vi "FillClassFamTree.vi"(7 "référence":refnum<vi>, 8 "ErrorIn(No Error)":errorcluster caption="entrée d'erreur (pas d'erreur)", 9 "LdClassArr":string[](array[string]), 10 "LdNameArr":string[](array[string]), 11 "SelectedClass":string) -> (0 "sortie d'erreur":errorcluster, 1 "Text":string[][](array[string]), 2 "Functions":string[][](array[string]), 3 "Classes":string[][](array[string]))   [LabVIEW 2019]
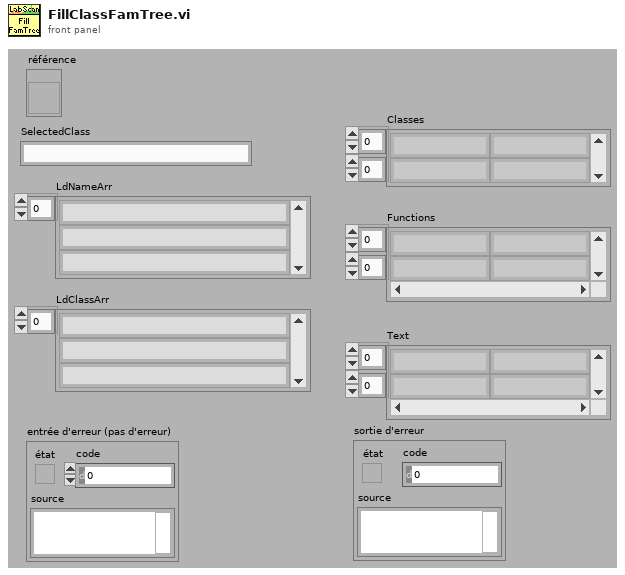
[diagram p1: front panel]
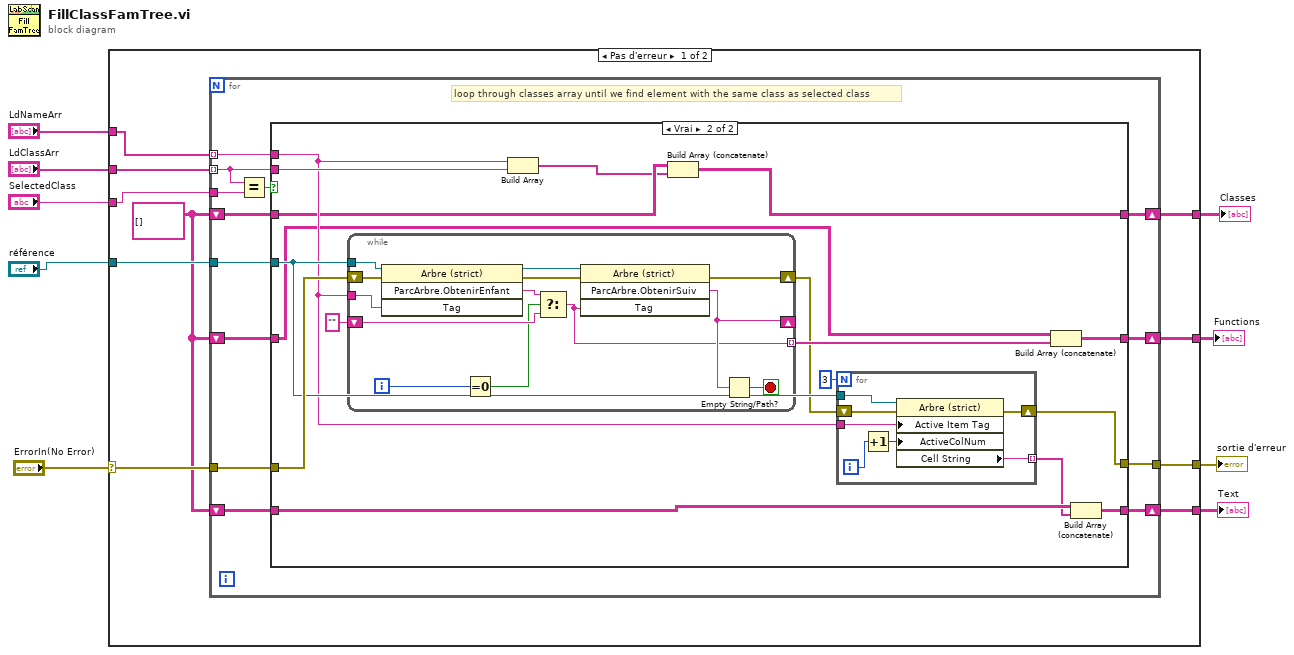
[diagram p0: block diagram]
diagram:
  n1 = case shown="Pas d'erreur" "ErrorIn(No Error)" {
    selector: "ErrorIn(No Error)" -> [w11 w74]
    tunnel: "LdNameArr" -> [w19 _]
    tunnel: "LdClassArr" -> [w18 _]
    tunnel: "SelectedClass" -> [w17 _]
    tunnel: [w16 w74] -> w6
    tunnel: [w15 _] -> w5
    tunnel: "référence" -> [w14 _]
    tunnel: [w13 _] -> w3
    tunnel: [w12 _] -> w2
    frame No Error {
      w10 = string[][] []
      n2 = for {
        tunnel: w18 -> [w30] mode=indexing
        tunnel: w17 -> [w32]
        shift-right: [w29] -> w15
        shift-left: w10 -> [w28]
        tunnel: w19 -> [w25] mode=indexing
        tunnel: [w24] -> w16
        tunnel: w14 -> [w23]
        tunnel: w11 -> [w22]
        shift-right: [w27] -> w13
        shift-left: w10 -> [w21]
        shift-right: [w26] -> w12
        shift-left: w10 -> [w20]
        # "loop through classes array until we find element with the same class as selected class"
        n3 = Equal?(x=w30, y=w32) -> (x = y?=w31:bool)
        n4 = case shown="Vrai" w31 {
          tunnel: w30 -> [_ w51]
          tunnel: [w36 w53] -> w29
          tunnel: w28 -> [w36 w40]
          tunnel: [w34 w43] -> w27
          tunnel: [w33 w46] -> w26
          tunnel: w25 -> [_ w48]
          tunnel: w22 -> [w35 w50]
          tunnel: [w35 w37] -> w24
          tunnel: w23 -> [_ w49]
          tunnel: w21 -> [w34 w42]
          tunnel: w20 -> [w33 w45]
          frame False {
            # "not the selected class"
          }
          frame True {
            n5 = while {
              shift-right: [w63] -> w38
              shift-left: w50 -> [w65]
              tunnel: w48 -> [w61]
              tunnel: w49 -> [w55]
              shift-right: [w56] -> _
              shift-left: "" ("Navigate Tree:Get Next Item") -> [w59]
              tunnel: [w54] -> w41 mode=indexing
              i -> [w60]
              stop <- w66 stop-if-true
              n6 = invoke on="Nœud de méthode" class="Arbre (strict)" method="ParcArbre.ObtenirEnfant"(reference=w55, error in=w65, "Tag"=w61) -> (reference out=w62:refnum<vi>, error out=w64:errorcluster, "Navigate Tree:Get Child"=w57:string)  [unwired: 1 in, 1 out]
              n7 = Equal To 0?(x=w60) -> (x = 0?=w58:bool)
              n8 = Select(t=w57, s=w58, f=w59) -> (s? t:f=w54:string)
              n9 = invoke on="Nœud de méthode" class="Arbre (strict)" method="ParcArbre.ObtenirSuiv"(reference=w62, error in=w64, "Tag"=w54) -> (error out=w63:errorcluster, "Navigate Tree:Get Next Item"=w56:string)  [unwired: 1 in, 2 out]
              n10 = Empty String/Path?(string/path=w56) -> (empty?=w66:bool)
            }
            n11 = Build Array(w48, w51) -> (w39:string[])
            n12 = Build Array (concatenate)(w40, w39) -> (w53:string[][])
            n13 = for {
              N: 3 -> [_]
              tunnel: w48 -> [w73]
              tunnel: [w70] -> w44 mode=indexing
              tunnel: w49 -> [w68]
              shift-right: [w69] -> w37
              shift-left: w38 -> [w67]
              i -> [w72]
              n14 = Increment(x=w72) -> (x+1=w71:i32)
              n15 = property on="Nœud de propriété" class="Arbre (strict)"(reference=w68, error in=w67, "Active Item Tag"=w73, "ActiveColNum"=w71) -> (error out=w69:errorcluster, "Cell String"=w70:string)  [unwired: 1 out]
            }
            n16 = Build Array (concatenate)(w42, w41) -> (w43:string[][])
            n17 = Build Array (concatenate)(w45, w44) -> (w46:string[][])
          }
        }
      }
    }
    frame Error {
    }
  }
  "sortie d'erreur" <- w6
  "Classes" <- w5
  "Functions" <- w3
  "Text" <- w2
